vi "GetFunctionalGlobalVisFromProject.vi"() -> ()   [LabVIEW 2020]
panel:
  out "Functional Global Variables in Active Project":string
  # "This tool is used for documenting the functional global variables (FGV) in a project.\n\n- Open the prject you want to document\n- Run the VI\n- Check the output in markdown format"
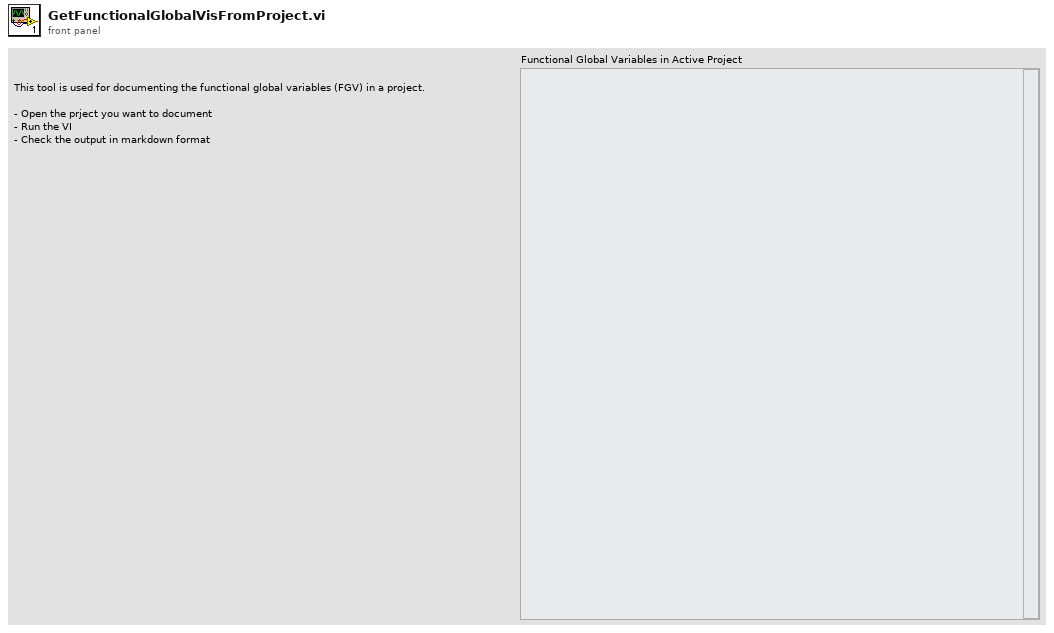
[diagram p1: front panel]
types:
  T1 = enum32{"invalid VI type", "Standard VI", "Control VI", "Global VI", "Polymorphic VI", "Configuration VI", "SubSystem", "Facade VI", "Method VI", "Statechart Diagram VI"}
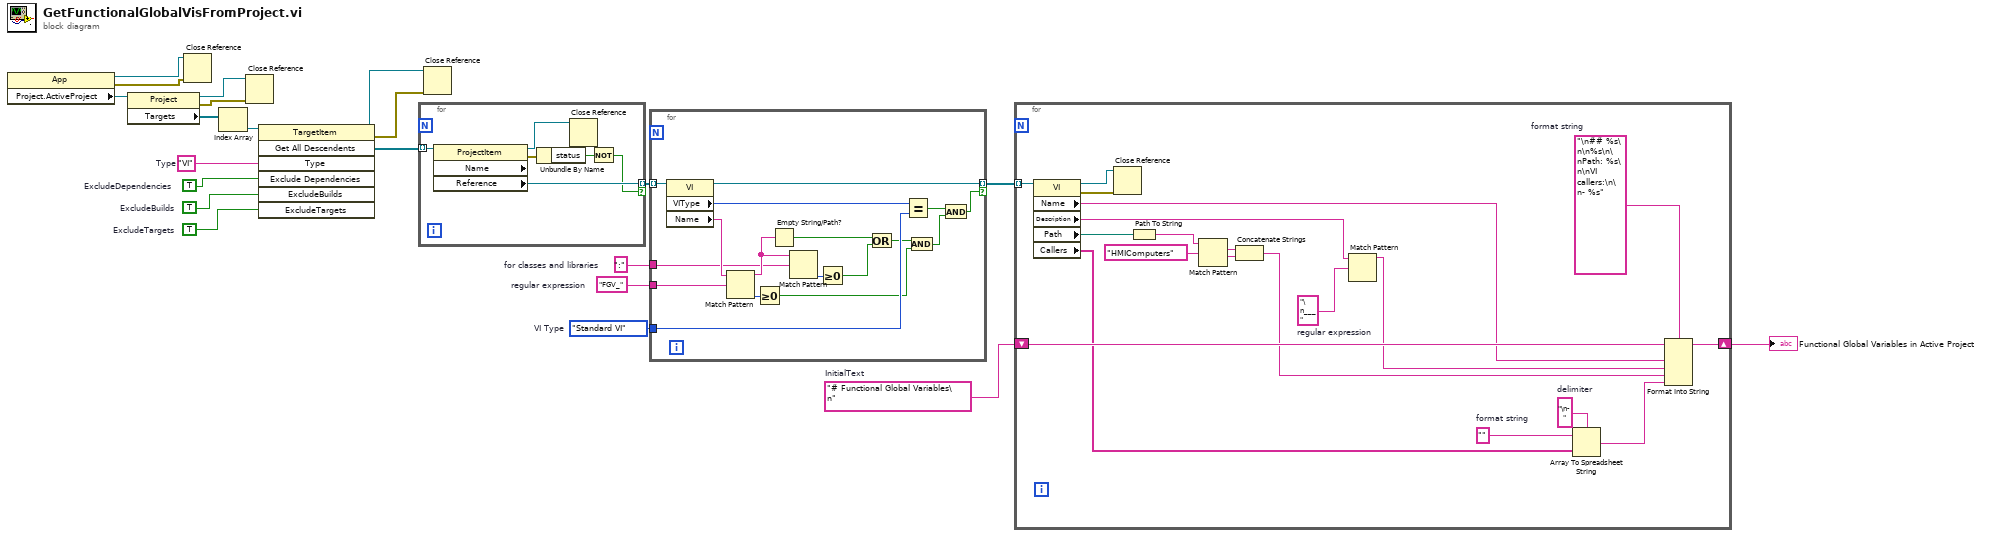
[diagram p0: block diagram]
diagram:
  w1 = ":"  # for classes and libraries
  w4 = "# Functional Global Variables\n"  # InitialText
  w5 = "FGV_"  # regular expression
  w12 = T1."Standard VI"  # VI Type
  w15 = "VI"  # Type
  w16 = TRUE  # ExcludeTargets
  w17 = TRUE  # ExcludeBuilds
  w18 = TRUE  # ExcludeDependencies
  n1 = property class="App"() -> (reference out=w11:refnum<vi>, error out=w10:errorcluster, "Project.ActiveProject"=w20:refnum<vi>)  [unwired: 2 in]
  n2 = property class="Project"(reference=w20) -> (reference out=w8:refnum<vi>, error out=w9:errorcluster, "Targets"=w21:refnum<vi>[])  [unwired: 1 in]
  n3 = Close Reference(reference=w11, error in (no error)=w10) -> ()  [unwired: 1 out]
  n4 = Index Array(array=w21) -> (element=w19:refnum<vi>)  [unwired: 1 in]
  n5 = Close Reference(reference=w8, error in (no error)=w9) -> ()  [unwired: 1 out]
  n6 = invoke class="TargetItem" method="Get All Descendents"(reference=w19, "Type"=w15, "Exclude Dependencies"=w18, "ExcludeBuilds"=w17, "ExcludeTargets"=w16) -> (reference out=w6:refnum<vi>, error out=w7:errorcluster, "All Descendents"=w14:refnum<vi>[])  [unwired: 2 in, 4 out]
  n7 = for {
    tunnel: w14 -> [w27] mode=indexing
    tunnel: [w26] -> w13 mode=indexing if=w23
    n8 = property class="ProjectItem" props=["Name", "Reference"](reference=w27) -> (reference out=w22:refnum<vi>, error out=w25:errorcluster, "Reference"=w26:refnum<vi>)  [unwired: 1 in, 1 out]
    n9 = Unbundle By Name(w25) -> ("status"=w24:bool)
    n10 = Close Reference(reference=w22) -> ()  [unwired: 1 in, 1 out]
    n11 = Not(x=w24) -> (.not. x?=w23:bool)
  }
  n12 = Close Reference(reference=w6, error in (no error)=w7) -> ()  [unwired: 1 out]
  n13 = for {
    tunnel: w13 -> [w44] mode=indexing
    tunnel: [w41] -> w2 mode=indexing if=w36
    tunnel: w12 -> [w42]
    tunnel: w5 -> [w39]
    tunnel: w1 -> [w30]
    n14 = property class="VI"(reference=w44) -> (reference out=w41:refnum<vi>, "VIType"=w43:T1, "Name"=w40:string)  [unwired: 1 in, 1 out]
    n15 = Match Pattern(string=w40, regular expression=w39) -> (before substring=w31:string, offset past match=w38:i32)  [unwired: 1 in, 2 out]
    n16 = Greater Or Equal To 0?(x=w38) -> (x >= 0?=w28:bool)
    n17 = Empty String/Path?(string/path=w31) -> (empty?=w35:bool)
    n18 = Match Pattern(string=w31, regular expression=w30) -> (offset past match=w32:i32)  [unwired: 1 in, 3 out]
    n19 = Greater Or Equal To 0?(x=w32) -> (x >= 0?=w29:bool)
    n20 = Or(x=w35, y=w29) -> (x .or. y?=w34:bool)
    n21 = Equal?(x=w43, y=w42) -> (x = y?=w37:bool)
    n22 = And(x=w34, y=w28) -> (x .and. y?=w33:bool)
    n23 = And(x=w37, y=w33) -> (x .and. y?=w36:bool)
  }
  n24 = for {
    tunnel: w2 -> [w64] mode=indexing
    shift-right: [w62] -> w3
    shift-left: w4 -> [w63]
    w46 = "\n___"  # regular expression
    w52 = ""  # format string
    w53 = "\n- "  # delimiter
    w61 = "\n## %s\n\n%s\n\nPath: %s\n\nVI callers:\n\n- %s"  # format string
    n25 = property class="VI"(reference=w64) -> (reference out=w50:refnum<vi>, error out=w51:errorcluster, "Name"=w49:string, "Description"=w47:string, "Path"=w55:path, "Callers"=w48:string[])  [unwired: 1 in]
    n26 = Close Reference(reference=w50, error in (no error)=w51) -> ()  [unwired: 1 out]
    n27 = Path To String(path=w55) -> (string=w59:string)
    n28 = Match Pattern(string=w59, regular expression="HMIComputers") -> (match substring=w57:string, after substring=w56:string)  [unwired: 1 in, 2 out]
    n29 = Concatenate Strings(w57, w56) -> (w54:string)
    n30 = Match Pattern(string=w47, regular expression=w46) -> (before substring=w45:string)  [unwired: 1 in, 3 out]
    n31 = Array To Spreadsheet String(delimiter (Tab)=w53, array=w48, 3:w52) -> (spreadsheet string=w60:string)
    n32 = Format Into String(format string=w61, initial string=w63, w49, w45, w54, w60) -> (resulting string=w62:string)  [unwired: 1 in, 1 out]
  }
  "Functional Global Variables in Active Project" <- w3
